vi "WKLXF25 St 60 Manual PLC Data 2.0.vi"(9 "station plc read string tags":T1={"Serial Number"={"Tag Name"="S060.PXI.Signals.PlltData.SN", "Network Path"="172.15.51.1,1,0", "use opc"=FALSE, "DataSocket Reference"={"CWDSLib._DCWDataSocket"=refnum, "CWDSLib._DCWData"=refnum, "OnDataUpdated"=0, "OnStatusUpdated"=0}}, "Pallet Number"={"Tag Name"="S060.PXI.Signals.PlltData.SN", "Network Path"="172.15.51.1,1,0", "use opc"=FALSE, "DataSocket Reference"={"CWDSLib._DCWDataSocket"=refnum, "CWDSLib._DCWData"=refnum, "OnDataUpdated"=0, "OnStatusUpdated"=0}}, "Inalfa Part Number"={"Tag Name"="S060.PXI.Signals.PlltData.SN", "Network Path"="172.15.51.1,1,0", "use opc"=FALSE, "DataSocket Reference"={"CWDSLib._DCWDataSocket"=refnum, "CWDSLib._DCWData"=refnum, "OnDataUpdated"=0, "OnStatusUpdated"=0}}, "Shade Color"={"Tag Name"="S060.PXI.Signals.PlltData.SN", "Network Path"="172.15.51.1,1,0", "use opc"=FALSE, "DataSocket Reference"={"CWDSLib._DCWDataSocket"=refnum, "CWDSLib._DCWData"=refnum, "OnDataUpdated"=0, "OnStatusUpdated"=0}}, "Model Type"={"Tag Name"="S060.PXI.Signals.PlltData.SN", "Network Path"="172.15.51.1,1,0", "use opc"=FALSE, "DataSocket Reference"={"CWDSLib._DCWDataSocket"=refnum, "CWDSLib._DCWData"=refnum, "OnDataUpdated"=0, "OnStatusUpdated"=0}}, "Customer Number"={"Tag Name"="S060.PXI.Signals.PlltData.SN", "Network Path"="172.15.51.1,1,0", "use opc"=FALSE, "DataSocket Reference"={"CWDSLib._DCWDataSocket"=refnum, "CWDSLib._DCWData"=refnum, "OnDataUpdated"=0, "OnStatusUpdated"=0}}, "Part History Number"={"Tag Name"="S060.PXI.Signals.PlltData.SN", "Network Path"="172.15.51.1,1,0", "use opc"=FALSE, "DataSocket Reference"={"CWDSLib._DCWDataSocket"=refnum, "CWDSLib._DCWData"=refnum, "OnDataUpdated"=0, "OnStatusUpdated"=0}}, "Shade 1 Barcode"={"Tag Name"="S060.PXI.Signals.PlltData.SN", "Network Path"="172.15.51.1,1,0", "use opc"=FALSE, "DataSocket Reference"={"CWDSLib._DCWDataSocket"=refnum, "CWDSLib._DCWData"=refnum, "OnDataUpdated"=0, "OnStatusUpdated"=0}}, "Shade 2 Barcode"={"Tag Name"="S060.PXI.Signals.PlltData.SN", "Network Path"="172.15.51.1,1,0", "use opc"=FALSE, "DataSocket Reference"={"CWDSLib._DCWDataSocket"=refnum, "CWDSLib._DCWData"=refnum, "OnDataUpdated"=0, "OnStatusUpdated"=0}}, "Manual Serial Number"={"Tag Name"="S060.PXI.Signals.PlltData.SN", "Network Path"="172.15.51.1,1,0", "use opc"=FALSE, "DataSocket Reference"={"CWDSLib._DCWDataSocket"=refnum, "CWDSLib._DCWData"=refnum, "OnDataUpdated"=0, "OnStatusUpdated"=0}}, "Manual Inalfa Part Number"={"Tag Name"="S060.PXI.Signals.PlltData.SN", "Network Path"="172.15.51.1,1,0", "use opc"=FALSE, "DataSocket Reference"={"CWDSLib._DCWDataSocket"=refnum, "CWDSLib._DCWData"=refnum, "OnDataUpdated"=0, "OnStatusUpdated"=0}}, "Manual Shade Color"={"Tag Name"="S060.PXI.Signals.PlltData.SN", "Network Path"="172.15.51.1,1,0", "use opc"=FALSE, "DataSocket Reference"={"CWDSLib._DCWDataSocket"=refnum, "CWDSLib._DCWData"=refnum, "OnDataUpdated"=0, "OnStatusUpdated"=0}}, "Manual Model Type"={"Tag Name"="S060.PXI.Signals.PlltData.SN", "Network Path"="172.15.51.1,1,0", "use opc"=FALSE, "DataSocket Reference"={"CWDSLib._DCWDataSocket"=refnum, "CWDSLib._DCWData"=refnum, "OnDataUpdated"=0, "OnStatusUpdated"=0}}, "Manual Customer Number"={"Tag Name"="S060.PXI.Signals.PlltData.SN", "Network Path"="172.15.51.1,1,0", "use opc"=FALSE, "DataSocket Reference"={"CWDSLib._DCWDataSocket"=refnum, "CWDSLib._DCWData"=refnum, "OnDataUpdated"=0, "OnStatusUpdated"=0}}, "Manual Part History Number"={"Tag Name"="S060.PXI.Signals.PlltData.SN", "Network Path"="172.15.51.1,1,0", "use opc"=FALSE, "DataSocket Reference"={"CWDSLib._DCWDataSocket"=refnum, "CWDSLib._DCWData"=refnum, "OnDataUpdated"=0, "OnStatusUpdated"=0}}, "iGPS SN 0"={"Tag Name"="S060.PXI.Signals.PlltData.SN", "Network Path"="172.15.51.1,1,0", "use opc"=FALSE, "DataSocket Reference"={"CWDSLib._DCWDataSocket"=refnum, "CWDSLib._DCWData"=refnum, "OnDataUpdated"=0, "OnStatusUpdated"=0}}, "iGPS SN 1"={"Tag Name"="S060.PXI.Signals.PlltData.SN", "Network Path"="172.15.51.1,1,0", "use opc"=FALSE, "DataSocket Reference"={"CWDSLib._DCWDataSocket"=refnum, "CWDSLib._DCWData"=refnum, "OnDataUpdated"=0, "OnStatusUpdated"=0}}, "iGPS SN 2"={"Tag Name"="S060.PXI.Signals.PlltData.SN", "Network Path"="172.15.51.1,1,0", "use opc"=FALSE, "DataSocket Reference"={"CWDSLib._DCWDataSocket"=refnum, "CWDSLib._DCWData"=refnum, "OnDataUpdated"=0, "OnStatusUpdated"=0}}, "iGPS SN 3"={"Tag Name"="S060.PXI.Signals.PlltData.SN", "Network Path"="172.15.51.1,1,0", "use opc"=FALSE, "DataSocket Reference"={"CWDSLib._DCWDataSocket"=refnum, "CWDSLib._DCWData"=refnum, "OnDataUpdated"=0, "OnStatusUpdated"=0}}, "iGPS SN 4"={"Tag Name"="S060.PXI.Signals.PlltData.SN", "Network Path"="172.15.51.1,1,0", "use opc"=FALSE, "DataSocket Reference"={"CWDSLib._DCWDataSocket"=refnum, "CWDSLib._DCWData"=refnum, "OnDataUpdated"=0, "OnStatusUpdated"=0}}, "iGPS SN 5"={"Tag Name"="S060.PXI.Signals.PlltData.SN", "Network Path"="172.15.51.1,1,0", "use opc"=FALSE, "DataSocket Reference"={"CWDSLib._DCWDataSocket"=refnum, "CWDSLib._DCWData"=refnum, "OnDataUpdated"=0, "OnStatusUpdated"=0}}, "iGPS SN 6"={"Tag Name"="S060.PXI.Signals.PlltData.SN", "Network Path"="172.15.51.1,1,0", "use opc"=FALSE, "DataSocket Reference"={"CWDSLib._DCWDataSocket"=refnum, "CWDSLib._DCWData"=refnum, "OnDataUpdated"=0, "OnStatusUpdated"=0}}, "iGPS SN 7"={"Tag Name"="S060.PXI.Signals.PlltData.SN", "Network Path"="172.15.51.1,1,0", "use opc"=FALSE, "DataSocket Reference"={"CWDSLib._DCWDataSocket"=refnum, "CWDSLib._DCWData"=refnum, "OnDataUpdated"=0, "OnStatusUpdated"=0}}, "iGPS SN 8"={"Tag Name"="S060.PXI.Signals.PlltData.SN", "Network Path"="172.15.51.1,1,0", "use opc"=FALSE, "DataSocket Reference"={"CWDSLib._DCWDataSocket"=refnum, "CWDSLib._DCWData"=refnum, "OnDataUpdated"=0, "OnStatusUpdated"=0}}, "iGPS SN 9"={"Tag Name"="S060.PXI.Signals.PlltData.SN", "Network Path"="172.15.51.1,1,0", "use opc"=FALSE, "DataSocket Reference"={"CWDSLib._DCWDataSocket"=refnum, "CWDSLib._DCWData"=refnum, "OnDataUpdated"=0, "OnStatusUpdated"=0}}} {"iGPS SN 9"."DataSocket Reference"."OnStatusUpdated" format="%.0x"; "iGPS SN 9"."DataSocket Reference"."OnDataUpdated" format="%.0x"; "iGPS SN 8"."DataSocket Reference"."OnStatusUpdated" format="%.0x"; "iGPS SN 8"."DataSocket Reference"."OnDataUpdated" format="%.0x"; "iGPS SN 7"."DataSocket Reference"."OnStatusUpdated" format="%.0x"; "iGPS SN 7"."DataSocket Reference"."OnDataUpdated" format="%.0x"; "iGPS SN 6"."DataSocket Reference"."OnStatusUpdated" format="%.0x"; "iGPS SN 6"."DataSocket Reference"."OnDataUpdated" format="%.0x"; "iGPS SN 5"."DataSocket Reference"."OnStatusUpdated" format="%.0x"; "iGPS SN 5"."DataSocket Reference"."OnDataUpdated" format="%.0x"; "iGPS SN 4"."DataSocket Reference"."OnStatusUpdated" format="%.0x"; "iGPS SN 4"."DataSocket Reference"."OnDataUpdated" format="%.0x"; "iGPS SN 3"."DataSocket Reference"."OnStatusUpdated" format="%.0x"; "iGPS SN 3"."DataSocket Reference"."OnDataUpdated" format="%.0x"; "iGPS SN 2"."DataSocket Reference"."OnStatusUpdated" format="%.0x"; "iGPS SN 2"."DataSocket Reference"."OnDataUpdated" format="%.0x"; "iGPS SN 1"."DataSocket Reference"."OnStatusUpdated" format="%.0x"; "iGPS SN 1"."DataSocket Reference"."OnDataUpdated" format="%.0x"; "iGPS SN 0"."DataSocket Reference"."OnStatusUpdated" format="%.0x"; "iGPS SN 0"."DataSocket Reference"."OnDataUpdated" format="%.0x"; "Manual Part History Number"."DataSocket Reference"."OnStatusUpdated" format="%.0x"; "Manual Part History Number"."DataSocket Reference"."OnDataUpdated" format="%.0x"; "Manual Customer Number"."DataSocket Reference"."OnStatusUpdated" format="%.0x"; "Manual Customer Number"."DataSocket Reference"."OnDataUpdated" format="%.0x"; "Manual Model Type"."DataSocket Reference"."OnStatusUpdated" format="%.0x"; "Manual Model Type"."DataSocket Reference"."OnDataUpdated" format="%.0x"; "Manual Shade Color"."DataSocket Reference"."OnStatusUpdated" format="%.0x"; "Manual Shade Color"."DataSocket Reference"."OnDataUpdated" format="%.0x"; "Manual Inalfa Part Number"."DataSocket Reference"."OnStatusUpdated" format="%.0x"; "Manual Inalfa Part Number"."DataSocket Reference"."OnDataUpdated" format="%.0x"; "Manual Serial Number"."DataSocket Reference"."OnStatusUpdated" format="%.0x"; "Manual Serial Number"."DataSocket Reference"."OnDataUpdated" format="%.0x"; "Shade 2 Barcode"."DataSocket Reference"."OnStatusUpdated" format="%.0x"; "Shade 2 Barcode"."DataSocket Reference"."OnDataUpdated" format="%.0x"; "Shade 1 Barcode"."DataSocket Reference"."OnStatusUpdated" format="%.0x"; "Shade 1 Barcode"."DataSocket Reference"."OnDataUpdated" format="%.0x"; "Part History Number"."DataSocket Reference"."OnStatusUpdated" format="%.0x"; "Part History Number"."DataSocket Reference"."OnDataUpdated" format="%.0x"; "Customer Number"."DataSocket Reference"."OnStatusUpdated" format="%.0x"; "Customer Number"."DataSocket Reference"."OnDataUpdated" format="%.0x"; "Model Type"."DataSocket Reference"."OnStatusUpdated" format="%.0x"; "Model Type"."DataSocket Reference"."OnDataUpdated" format="%.0x"; "Shade Color"."DataSocket Reference"."OnStatusUpdated" format="%.0x"; "Shade Color"."DataSocket Reference"."OnDataUpdated" format="%.0x"; "Inalfa Part Number"."DataSocket Reference"."OnStatusUpdated" format="%.0x"; "Inalfa Part Number"."DataSocket Reference"."OnDataUpdated" format="%.0x"; "Pallet Number"."DataSocket Reference"."OnStatusUpdated" format="%.0x"; "Pallet Number"."DataSocket Reference"."OnDataUpdated" format="%.0x"; "Serial Number"."DataSocket Reference"."OnStatusUpdated" format="%.0x"; "Serial Number"."DataSocket Reference"."OnDataUpdated" format="%.0x"}) -> (1 "No Data?":bool, 2 "Error String":string, 3 "PLC Data":T4)   [LabVIEW 2018]
uses:
  02.Type Def's/WKLXF25 St 60 PLC Data Control.ctl
  02.Type Def's/station plc read string tags.ctl
  05.UserVI's/type defs/plc path and tag.ctl
  <vilib>/Platform/dataskt.llb/DataSocket Reference Type.ctl
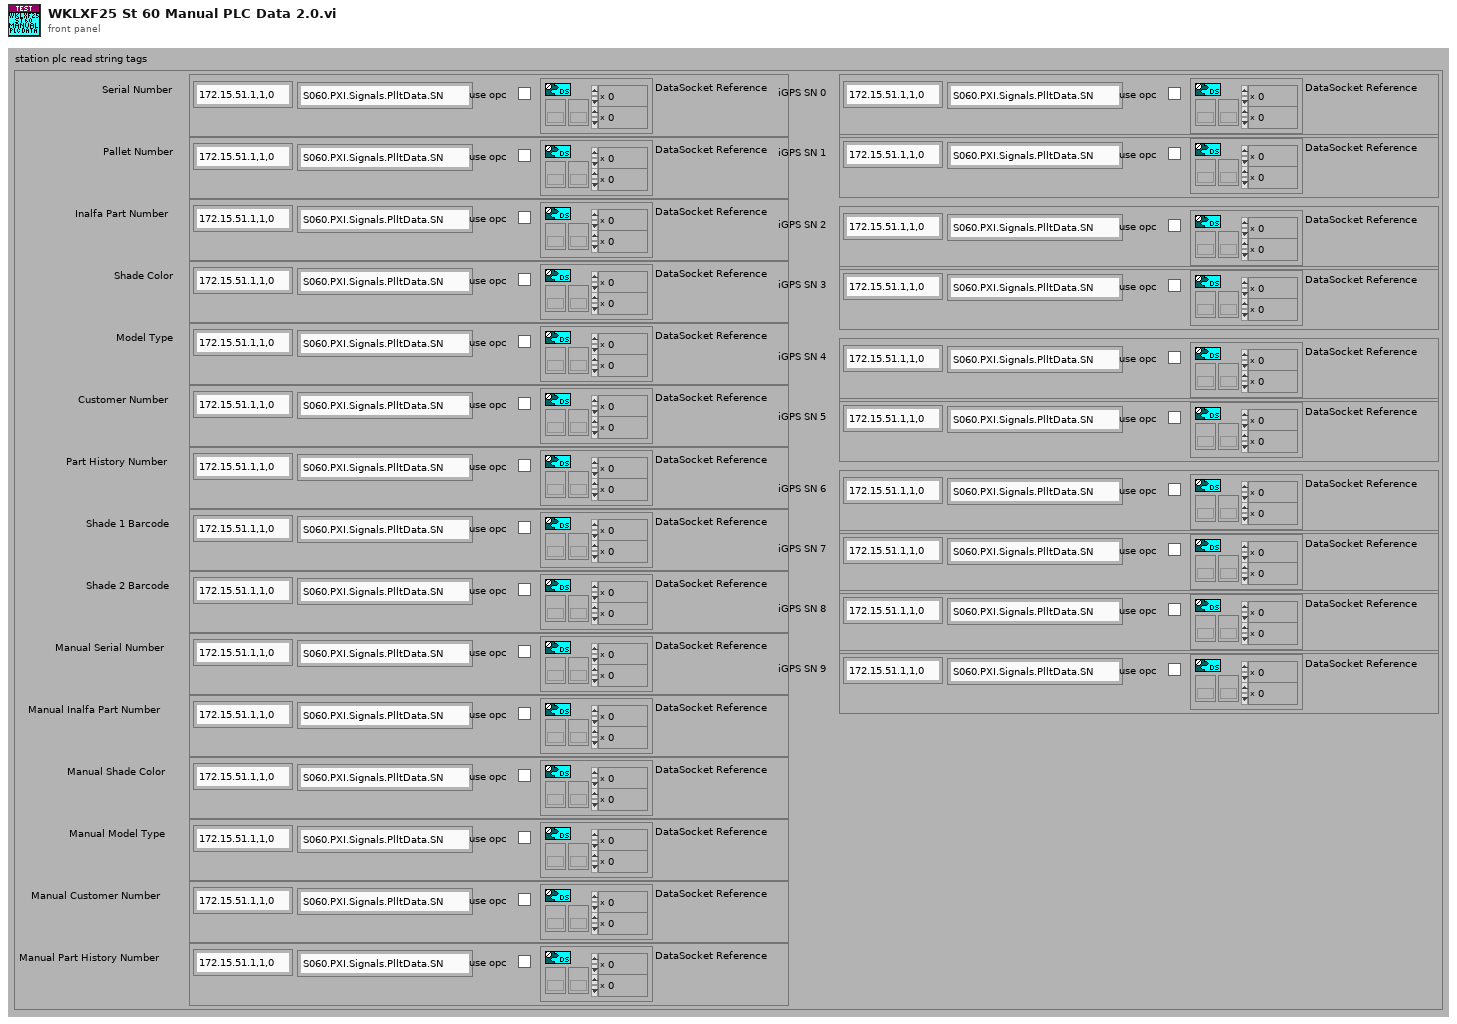
[diagram p1: front panel]
types:
  T1 = typedef "station plc read string tags.ctl" = cluster{"Serial Number":T2, "Pallet Number":T2, "Inalfa Part Number":T2, "Shade Color":T2, "Model Type":T2, "Customer Number":T2, "Part History Number":T2, "Shade 1 Barcode":T2, "Shade 2 Barcode":T2, "Manual Serial Number":T2, "Manual Inalfa Part Number":T2, "Manual Shade Color":T2, "Manual Model Type":T2, "Manual Customer Number":T2, "Manual Part History Number":T2, "iGPS SN 0":T2, "iGPS SN 1":T2, "iGPS SN 2":T2, "iGPS SN 3":T2, "iGPS SN 4":T2, "iGPS SN 5":T2, "iGPS SN 6":T2, "iGPS SN 7":T2, "iGPS SN 8":T2, "iGPS SN 9":T2}
  T2 = typedef "plc path and tag.ctl" = cluster{"Tag Name":string, "Network Path":string, "use opc":bool, "DataSocket Reference":T3}
  T3 = typedef "DataSocket Reference Type.ctl" = cluster{"CWDSLib._DCWDataSocket":refnum<k7>, "CWDSLib._DCWData":refnum<k7>, "OnDataUpdated":u32, "OnStatusUpdated":u32}
  T4 = typedef "WKLXF25 St 60 PLC Data Control.ctl" = cluster{"Serial Number":string, "Inalfa Part Number":string, "Sunshade Color":string, "Shade 1 Barcode":string, "Shade 2 Barcode":string, "Model Type":string, "Part History Number":string, "Customer Number":string}
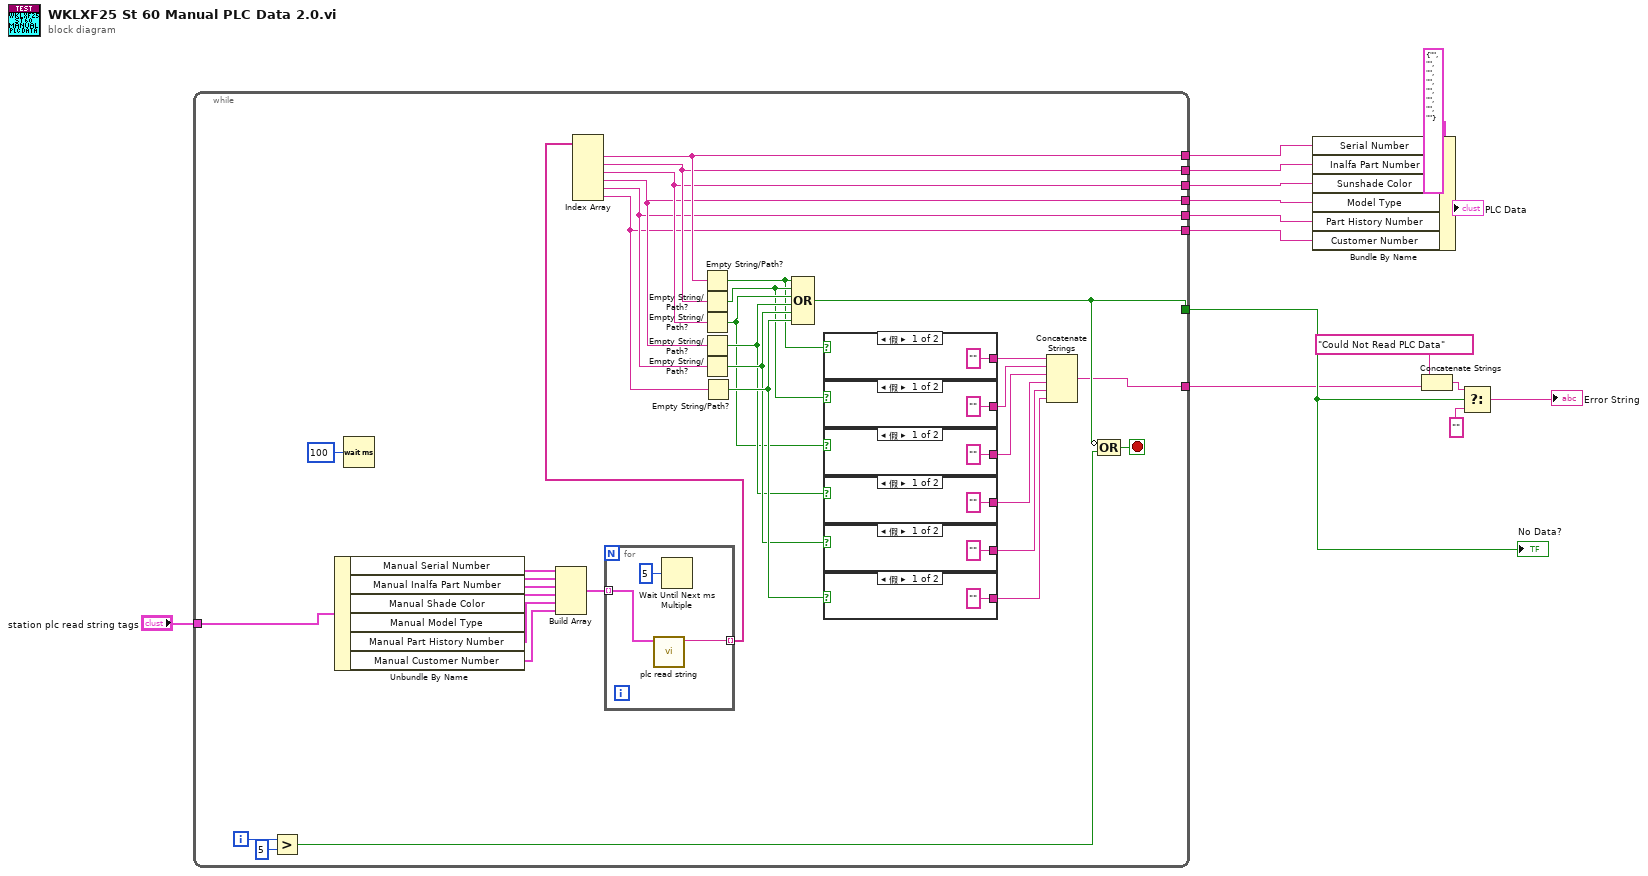
[diagram p0: block diagram]
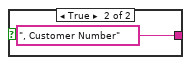
[diagram p2: hidden frame]
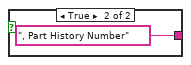
[diagram p3: hidden frame]
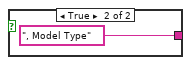
[diagram p4: hidden frame]
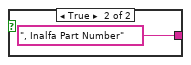
[diagram p5: hidden frame]
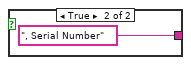
[diagram p6: hidden frame]
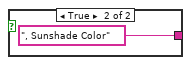
[diagram p7: hidden frame]
diagram:
  n1 = while {
    tunnel: [w44] -> w15
    tunnel: [w43] -> w10
    tunnel: [w42] -> w9
    tunnel: [w41] -> w8
    tunnel: [w27] -> w7
    tunnel: [w26] -> w6
    tunnel: [w25] -> w5
    tunnel: [w28] -> w2
    tunnel: "station plc read string tags" -> [w17]
    i -> [w48]
    stop <- w45 stop-if-true
    n2 = Greater?(x=w48, y=5) -> (0:w46:bool)
    n3 = Unbundle By Name(w17) -> ("Manual Serial Number"=w18:T2, "Manual Inalfa Part Number"=w19:T2, "Manual Shade Color"=w20:T2, "Manual Model Type"=w21:T2, "Manual Part History Number"=w22:T2, "Manual Customer Number"=w23:T2)
    n4 = Wait (ms)(milliseconds to wait=u32 100) -> ()  [unwired: 1 out]
    n5 = Build Array(w18, w19, w20, w21, w22, w23) -> (w24:T2[])
    n6 = for {
      tunnel: w24 -> [w52] mode=indexing
      tunnel: [w51] -> w16 mode=indexing
      n7 = call "plc read string.vi"("addr,tag"=w52) -> ("Data"=w51:string)  [unwired: 9 in, 1 out]
      n8 = Wait Until Next ms Multiple(millisecond multiple=u32 5) -> ()  [unwired: 1 out]
    }
    n9 = Index Array(array=w16) -> (element #1=w43:string, element #2=w42:string, element #3=w41:string, element #4=w27:string, element #5=w26:string, element #6=w25:string)  [unwired: 6 in]
    n10 = Empty String/Path?(string/path=w43) -> (empty?=w35:bool)
    n11 = Empty String/Path?(string/path=w42) -> (empty?=w36:bool)
    n12 = Empty String/Path?(string/path=w41) -> (empty?=w37:bool)
    n13 = Empty String/Path?(string/path=w27) -> (empty?=w38:bool)
    n14 = Empty String/Path?(string/path=w26) -> (empty?=w39:bool)
    n15 = Empty String/Path?(string/path=w25) -> (empty?=w40:bool)
    n16 = Compound Arithmetic op=OR(w35, w36, w37, w38, w39, w40) -> (w44:bool)
    n17 = case shown="假" w35 {
      tunnel: ["" ", Serial Number"] -> w34
      frame False {
      }
      frame True {
      }
    }
    n18 = case shown="假" w36 {
      tunnel: ["" ", Inalfa Part Number"] -> w33
      frame False {
      }
      frame True {
      }
    }
    n19 = case shown="假" w37 {
      tunnel: ["" ", Sunshade Color"] -> w32
      frame False {
      }
      frame True {
      }
    }
    n20 = case shown="假" w38 {
      tunnel: ["" ", Model Type"] -> w31
      frame False {
      }
      frame True {
      }
    }
    n21 = case shown="假" w39 {
      tunnel: ["" ", Part History Number"] -> w30
      frame False {
      }
      frame True {
      }
    }
    n22 = case shown="假" w40 {
      tunnel: ["" ", Customer Number"] -> w29
      frame False {
      }
      frame True {
      }
    }
    n23 = Concatenate Strings(w34, w33, w32, w31, w30, w29) -> (w28:string)
    n24 = Compound Arithmetic op=OR(invert w44, w46) -> (w45:bool)
  }
  "No Data?" <- w15
  n25 = Bundle By Name(cluster=T4 {"Serial Number"="", "Inalfa Part Number"="", "Sunshade Color"="", "Shade 1 Barcode"="", "Shade 2 Barcode"="", "Model Type"="", "Part History Number"="", "Customer Number"=""} ("St 60 PLC Data Control"), "Serial Number"=w10, "Inalfa Part Number"=w9, "Sunshade Color"=w8, "Model Type"=w7, "Part History Number"=w6, "Customer Number"=w5) -> (→"PLC Data":T4)
  n26 = Concatenate Strings("Could Not Read PLC Data" ("t"), w2) -> (w3:string)
  n27 = Select(t=w3, s=w15, f="") -> (s? t:f=→"Error String":string)
